vi "Vision Processing.vi"(4 "error in (no error)":errorcluster, 7 "Image Size":T3=enum."160x120") -> ()   [LabVIEW 2015]
doc: "This VI runs in parallel to other tasks. It gets images from the camera, processes them for color or shape and use that information to affect robot behavior."
uses:
  <vilib>/Rock Robotics/WPI/Camera/WPI_CameraImageSize.ctl
  <vilib>/Rock Robotics/WPI/Camera/WPI_CameraWhite Balance Values.ctl
  <vilib>/Rock Robotics/WPI/Camera/WPI_CameraExposure Values.ctl
  <vilib>/Rock Robotics/WPI/Camera/WPI_CameraFrameRate.ctl
  <vilib>/Rock Robotics/Network Tables/NT Read Number.vi
  Robot Global Data.vi
  <vilib>/vision/NI_Vision_Development_Module.lvlib
panel:
  in  "Blue or Luma or Val or Inten Range":cluster{"Lower value":i32, "Upper value":i32}={"Lower value"=0, "Upper value"=200}
  in  "Green or Sat Range":cluster{"Lower value":i32, "Upper value":i32}={"Lower value"=20, "Upper value"=230}
  in  "Red or Hue Range":cluster{"Lower value":i32, "Upper value":i32}={"Lower value"=150, "Upper value"=255}
  out "Image Dst Out 2":T1(plugin-control)
  in  "Operation":T2(ring)
  out "Particle Reports (Pixels)[0].Center of Mass":cluster{"X":dbl, "Y":dbl}={"X"=88.72549019607843, "Y"=42.09313725490196}
  out "Image Dst Out":T1(plugin-control)
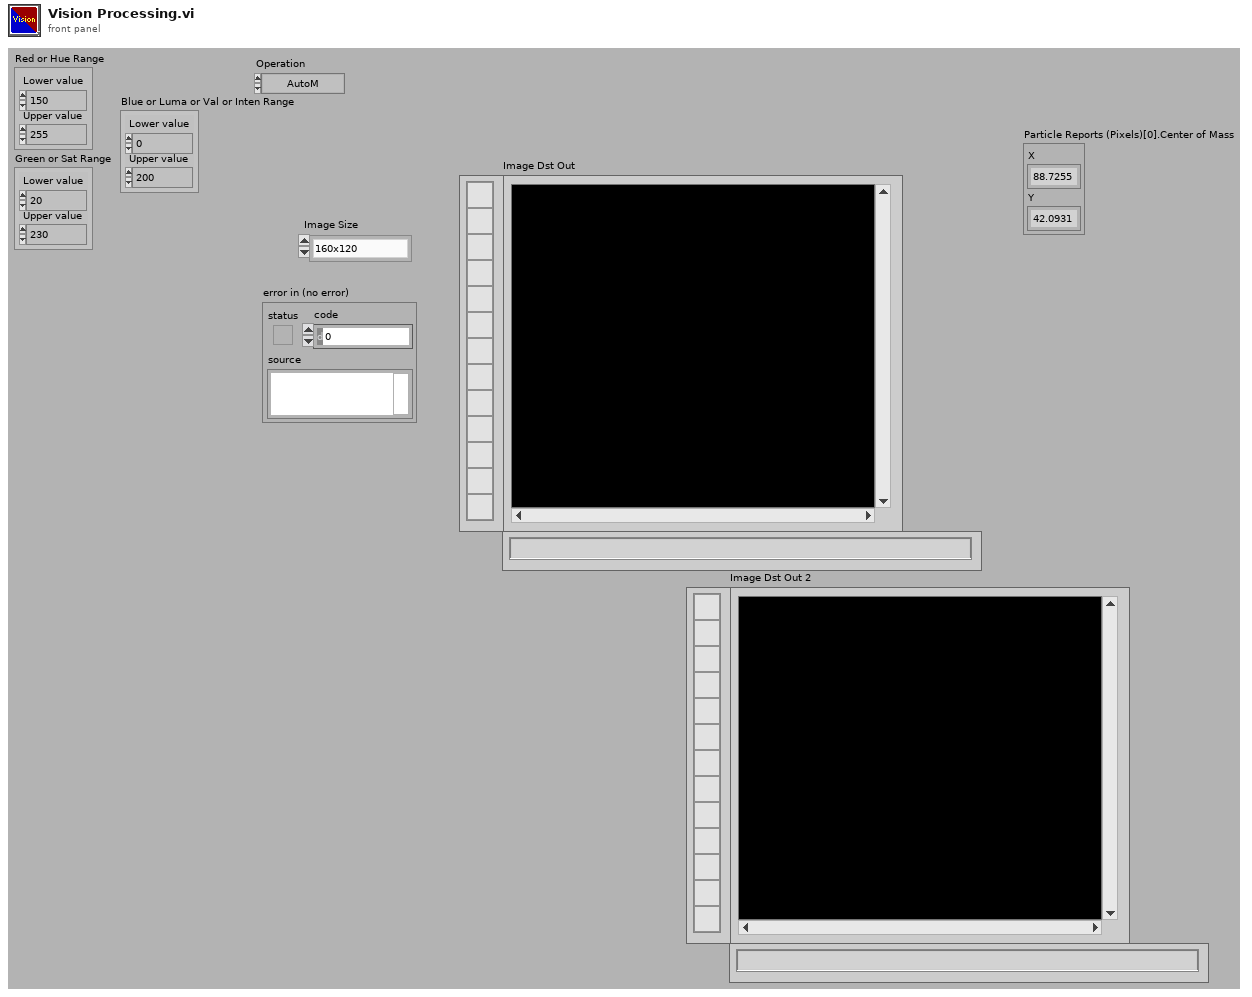
[diagram p1: front panel]
types:
  T1 = typedef "IMAQ Image.ctl" = refnum<image>
  T2 = enum32{"AutoM", "Close", "Dilate", "Erode", "Gradient", "Gradient out", "Gradient in", "Hit miss", "Open", "PClose", "POpen", "Thick", "Thin"}
  T3 = typedef "WPI_CameraImageSize.ctl" = enum16{"640x480", "320x240", "160x120", "Custom"}
  T4 = typedef "Image Type" = u32
  T5 = typedef "WPI_CameraFrameRate.ctl" = u32
  T6 = typedef "WPI_CameraExposure Values.ctl" = enum16{"Auto", "Flicker-free 50 Hz", "Flicker-free 60 Hz", "Hold current", "Custom"}
  T7 = typedef "WPI_CameraWhite Balance Values.ctl" = enum16{"Auto", "Fixed indoor", "Fixed outdoor 1", "Fixed outdoor 2", "Fixed fluorescent 1", "Fixed fluorescent 2", "Hold current", "Custom"}
  T8 = typedef "WPI_CameraDevRef.ctl" = cluster{"Camera Address":string, "CameraStatus":errorcluster}
  T9 = cluster{"Area":dbl, "Number of Holes":dbl, "Bounding Rect":cluster{"Left":dbl, "Top":dbl, "Right":dbl, "Bottom":dbl}, "Center of Mass":cluster{"X":dbl, "Y":dbl}, "Orientation":dbl, "Dimensions":cluster{"Width":dbl, "Height":dbl}}[]
  T10 = cluster{"Particle Reports (Pixels)[0]":cluster{"Area":dbl, "Number of Holes":dbl, "Bounding Rect":cluster{"Left":dbl, "Top":dbl, "Right":dbl, "Bottom":dbl}, "Center of Mass":cluster{"X":dbl, "Y":dbl}, "Orientation":dbl, "Dimensions":cluster{"Width":dbl, "Height":dbl}}, "Particle Reports (Pixels)[1]":cluster{"Area":dbl, "Number of Holes":dbl, "Bounding Rect":cluster{"Left":dbl, "Top":dbl, "Right":dbl, "Bottom":dbl}, "Center of Mass":cluster{"X":dbl, "Y":dbl}, "Orientation":dbl, "Dimensions":cluster{"Width":dbl, "Height":dbl}}, "Particle Reports (Pixels)[2]":cluster{"Area":dbl, "Number of Holes":dbl, "Bounding Rect":cluster{"Left":dbl, "Top":dbl, "Right":dbl, "Bottom":dbl}, "Center of Mass":cluster{"X":dbl, "Y":dbl}, "Orientation":dbl, "Dimensions":cluster{"Width":dbl, "Height":dbl}}, "Particle Reports (Pixels)[3]":cluster{"Area":dbl, "Number of Holes":dbl, "Bounding Rect":cluster{"Left":dbl, "Top":dbl, "Right":dbl, "Bottom":dbl}, "Center of Mass":cluster{"X":dbl, "Y":dbl}, "Orientation":dbl, "Dimensions":cluster{"Width":dbl, "Height":dbl}}, "Particle Reports (Pixels)[4]":cluster{"Area":dbl, "Number of Holes":dbl, "Bounding Rect":cluster{"Left":dbl, "Top":dbl, "Right":dbl, "Bottom":dbl}, "Center of Mass":cluster{"X":dbl, "Y":dbl}, "Orientation":dbl, "Dimensions":cluster{"Width":dbl, "Height":dbl}}, "Particle Reports (Pixels)[5]":cluster{"Area":dbl, "Number of Holes":dbl, "Bounding Rect":cluster{"Left":dbl, "Top":dbl, "Right":dbl, "Bottom":dbl}, "Center of Mass":cluster{"X":dbl, "Y":dbl}, "Orientation":dbl, "Dimensions":cluster{"Width":dbl, "Height":dbl}}, "Particle Reports (Pixels)[6]":cluster{"Area":dbl, "Number of Holes":dbl, "Bounding Rect":cluster{"Left":dbl, "Top":dbl, "Right":dbl, "Bottom":dbl}, "Center of Mass":cluster{"X":dbl, "Y":dbl}, "Orientation":dbl, "Dimensions":cluster{"Width":dbl, "Height":dbl}}, "Particle Reports (Pixels)[7]":cluster{"Area":dbl, "Number of Holes":dbl, "Bounding Rect":cluster{"Left":dbl, "Top":dbl, "Right":dbl, "Bottom":dbl}, "Center of Mass":cluster{"X":dbl, "Y":dbl}, "Orientation":dbl, "Dimensions":cluster{"Width":dbl, "Height":dbl}}, "Particle Reports (Pixels)[8]":cluster{"Area":dbl, "Number of Holes":dbl, "Bounding Rect":cluster{"Left":dbl, "Top":dbl, "Right":dbl, "Bottom":dbl}, "Center of Mass":cluster{"X":dbl, "Y":dbl}, "Orientation":dbl, "Dimensions":cluster{"Width":dbl, "Height":dbl}}}
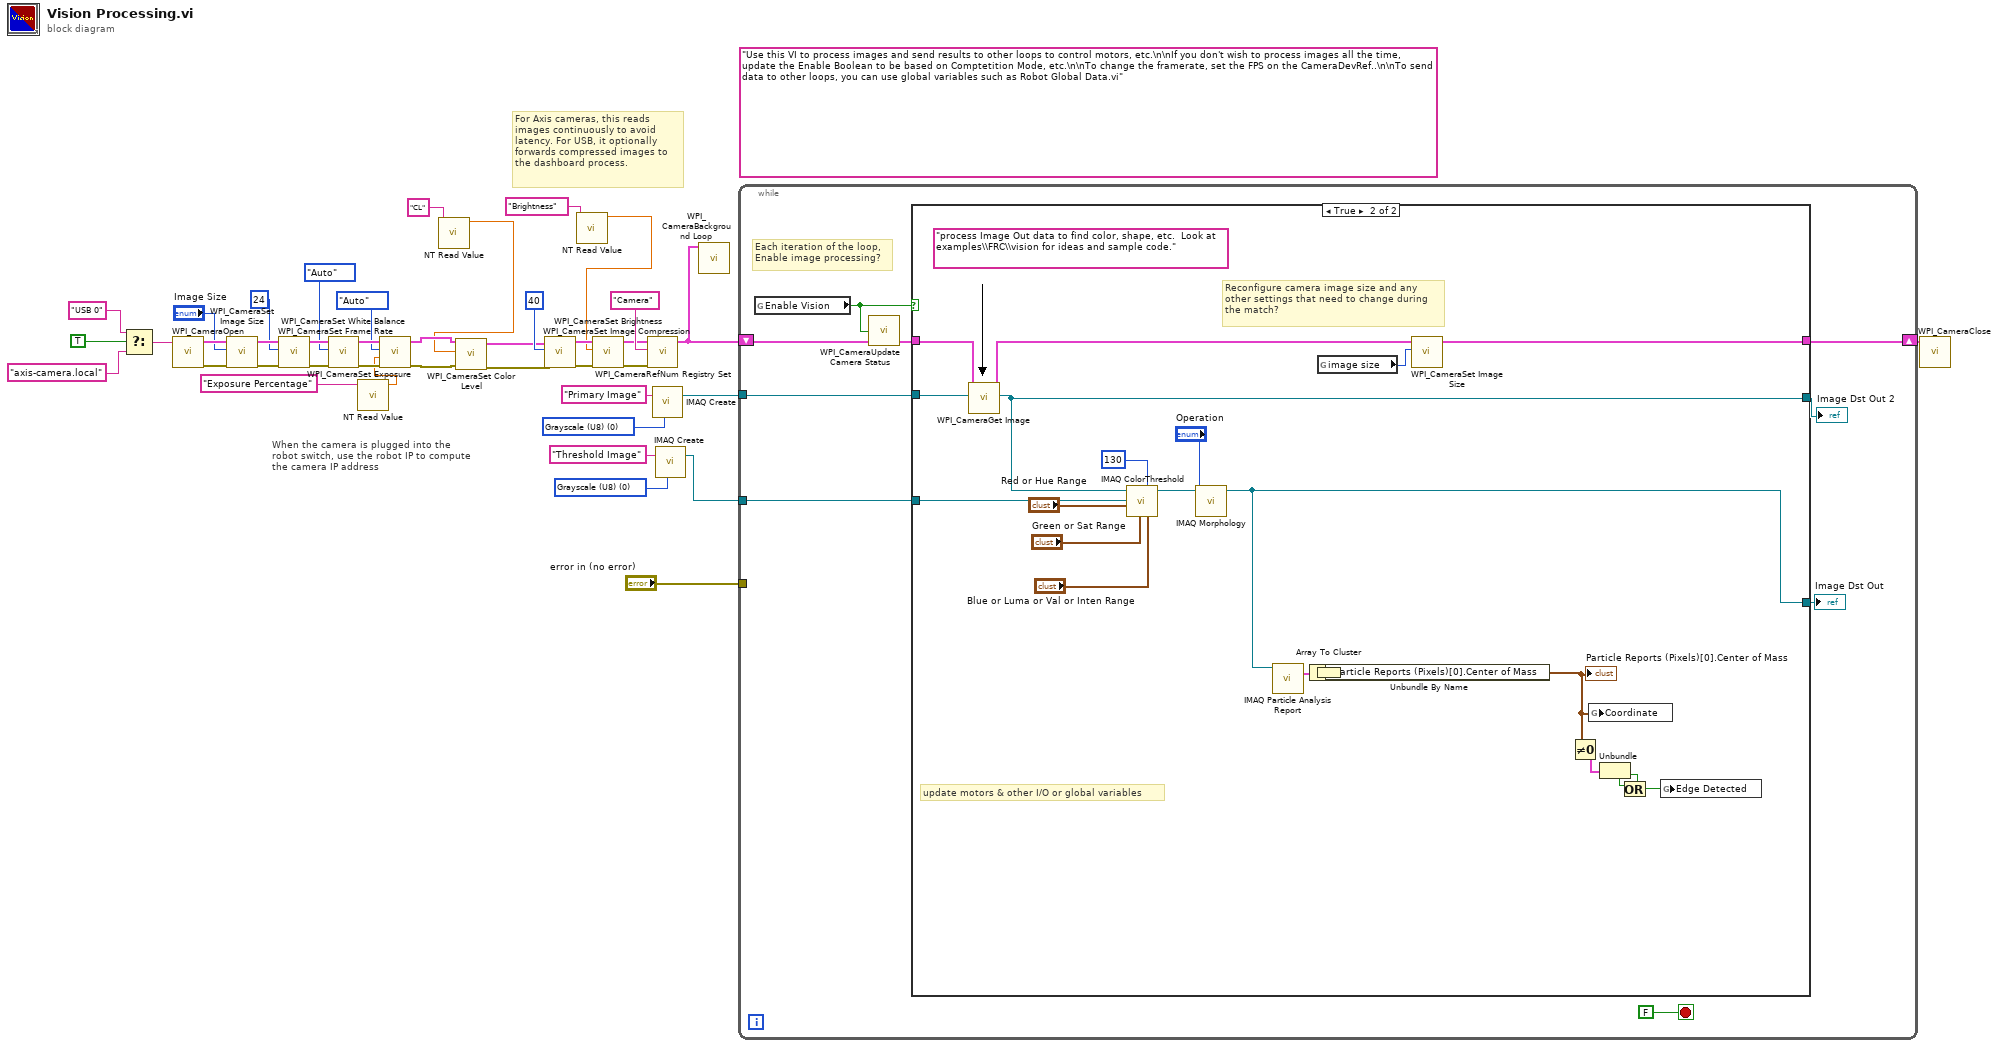
[diagram p0: block diagram]
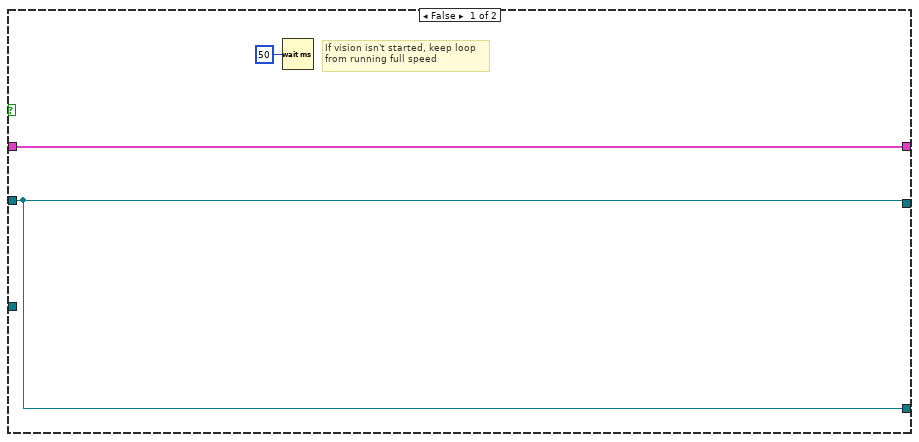
[diagram p2: hidden frame]
diagram:
  w13 = T4 0 items=["Grayscale (U8)", "Grayscale (I16)", "Grayscale (SGL)", "Complex (CSG)", "RGB (U32)", "HSL (U32)", "RGB (U64)", "Grayscale (U16)"] ("Image Type")
  (unwired) "Use this VI to process images and send results to other loops to control motors, etc.\n\nIf you don't wish to process images all the time, update the Enable Boolean to be based on Comptetition Mode, etc.\n\nTo change the framerate, set the FPS on the CameraDevRef..\n\nTo send data to other loops, you can use global variables such as Robot Global Data.vi"
  w41 = T4 0 items=["Grayscale (U8)", "Grayscale (I16)", "Grayscale (SGL)", "Complex (CSG)", "RGB (U32)", "HSL (U32)", "RGB (U64)"] ("Image Type")
  # "When the camera is plugged into the\nrobot switch, use the robot IP to compute\nthe camera IP address"
  # "For Axis cameras, this reads\nimages continuously to avoid\nlatency. For USB, it optionally\nforwards compressed images to\nthe dashboard process."
  n1 = Select(t="USB 0" ("format string"), s=TRUE ("dot notation? (F)"), f="axis-camera.local" ("format string")) -> (s? t:f=w15:string)
  n2 = call <vilib>:"WPI_CameraOpen.vi"("Camera Address"=w15) -> ("error out"=w31:errorcluster, "CameraDevRef"=w32:T8)  [unwired: 1 in, 8 out]
  n3 = call <vilib>:"WPI_CameraSet Image Size.vi"("error in (no error)"=w31, "Image Size"="Image Size", "CameraDevRef"=w32) -> ("error out"=w30:errorcluster, "CameraDevRef Out"=w33:T8)  [unwired: 1 in, 6 out]
  n4 = call <vilib>:"WPI_CameraSet Frame Rate.vi"("error in (no error)"=w30, "Frame Rate (fps)"=T5 24, "CameraDevRef"=w33) -> ("error out"=w29:errorcluster, "CameraDevRef Out"=w35:T8)  [unwired: 7 out]
  n5 = call <vilib>:"WPI_CameraSet White Balance.vi"("error in (no error)"=w29, "White Balance"=WPI_CameraWhite_Balance_Values."Auto", "CameraDevRef"=w35) -> ("error out"=w28:errorcluster, "CameraDevRef Out"=w34:T8)  [unwired: 1 in, 6 out]
  n6 = call-poly <vilib>:"NT Read Value.vi"("Name"="Exposure Percentage") -> ("Numeric"=w2:dbl)  [unwired: 9 in, 1 out]
  n7 = call <vilib>:"WPI_CameraSet Exposure.vi"("error in (no error)"=w28, "Exposure (%)"=w2, "Exposure"=WPI_CameraExposure_Values."Auto", "CameraDevRef"=w34) -> ("error out"=w9:errorcluster, "CameraDevRef Out"=w10:T8)  [unwired: 6 out]
  n8 = call-poly <vilib>:"NT Read Value.vi"("Name"="CL") -> ("Numeric"=w5:dbl)  [unwired: 9 in, 1 out]
  n9 = call <vilib>:"WPI_CameraSet Color Level.vi"("error in (no error)"=w9, "Color Level"=w5, "CameraDevRef"=w10) -> ("error out"=w7:errorcluster, "CameraDevRef Out"=w8:T8)  [unwired: 7 in]
  n10 = call <vilib>:"WPI_CameraSet Image Compression.vi"("error in (no error)"=w7, "Compression"=40, "CameraDevRef"=w8) -> ("error out"=w27:errorcluster, "CameraDevRef Out"=w36:T8)  [unwired: 7 out]
  n11 = call-poly <vilib>:"NT Read Value.vi"("Name"="Brightness") -> ("Numeric"=w4:dbl)  [unwired: 9 in, 1 out]
  n12 = call <vilib>:"WPI_CameraSet Brightness.vi"("error in (no error)"=w27, "Brightness"=w4, "CameraDevRef"=w36) -> ("error out"=w25:errorcluster, "CameraDevRef Out"=w26:T8)  [unwired: 7 out]
  n13 = call <vilib>:"WPI_CameraRefNum Registry Set.vi"("error in (no error)"=w25, "refnum name"="Camera", "CameraDevRef"=w26) -> ("CameraDevRef"=w21:T8)  [unwired: 1 in, 7 out]
  n14 = call "IMAQ Create"("Image Name"="Primary Image", "Image Type"=w41) -> ("New Image"=w39:T1)  [unwired: 2 in, 2 out]
  n15 = call "IMAQ Create"("Image Name"="Threshold Image", "Image Type"=w13) -> ("New Image"=w11:T1)  [unwired: 3 in, 1 out]
  n16 = call <vilib>:"WPI_CameraBackground Loop.vi"("CameraDevRef"=w21) -> ()  [unwired: 11 in]
  n17 = while {
    shift-right: [w49] -> w19
    shift-left: w21 -> [w47]
    tunnel: w39 -> [w48]
    tunnel: "error in (no error)" -> [_]
    tunnel: w11 -> [w44]
    stop <- FALSE stop-if-true
    # "Each iteration of the loop,\nEnable image processing?"
    n18 = global read "Robot Global Data.vi" "Enable Vision"() -> (w45:bool)
    n19 = call <vilib>:"WPI_CameraUpdate Camera Status.vi"("CameraDevRef In"=w47, "Enable Vision"=w45) -> ("CameraDevRef Out"=w46:T8)  [unwired: 3 in]
    n20 = case shown="True" w45 {
      tunnel: w48 -> [w51 w73]
      tunnel: [w53 w74] -> w49
      tunnel: w46 -> [w53 w71]
      tunnel: w44 -> [_ w69]
      tunnel: [w51 w59] -> w43
      tunnel: [w51 w57] -> w42
      frame False {
        # "If vision isn't started, keep loop\nfrom running full speed"
        n21 = Wait (ms)(milliseconds to wait=u32 50) -> ()  [unwired: 1 out]
      }
      frame True {
        (unwired) "process Image Out data to find color, shape, etc.  Look at examples\\FRC\\vision for ideas and sample code."
        # "update motors & other I/O or global variables"
        # "Reconfigure camera image size and any\nother settings that need to change during\nthe match?"
        n22 = call <vilib>:"WPI_CameraGet Image.vi"("Image"=w73, "CameraDevRef"=w71) -> ("Image Out"=w57:T1, "CameraDevRef Out"=w70:T8)  [unwired: 1 in, 7 out]
        n23 = call "IMAQ ColorThreshold"("Blue or Luma or Val or Inten Range"="Blue or Luma or Val or Inten Range", "Replace Value"=130, "Green or Sat Range"="Green or Sat Range", "Red or Hue Range"="Red or Hue Range", "Image Dst"=w69, "Image Src"=w57) -> ("Image Dst Out"=w60:T1)  [unwired: 4 in, 1 out]
        n24 = call "IMAQ Morphology"("Operation"="Operation", "Image Src"=w60) -> ("Image Dst Out"=w59:T1)  [unwired: 8 in, 1 out]
        n25 = call "IMAQ Particle Analysis Report"("Image"=w59) -> ("Particle Reports (Pixels)"=w67:T9)  [unwired: 5 in, 5 out]
        n26 = Array To Cluster(array=w67) -> (cluster=w66:T10)
        n27 = Unbundle By Name(w66) -> ("Particle Reports (Pixels)[0].Center of Mass"=w65:cluster{"X":dbl, "Y":dbl})
        "Particle Reports (Pixels)[0].Center of Mass" <- w65
        n28 = global read "Robot Global Data.vi" "image size"() -> (w72:T3)
        n29 = call <vilib>:"WPI_CameraSet Image Size.vi"("Image Size"=w72, "CameraDevRef"=w70) -> ("CameraDevRef Out"=w74:T8)  [unwired: 2 in, 7 out]
        n30 = Not Equal To 0?(x=w65) -> (x != 0?=w64:cluster{"X":bool, "Y":bool})
        n31 = global write "Robot Global Data.vi" "Coordinate"(w65) -> ()
        n32 = Unbundle(w64) -> ("X"=w63:bool, "Y"=w62:bool)
        n33 = Or(x=w63, y=w62) -> (x .or. y?=w61:bool)
        n34 = global write "Robot Global Data.vi" "Edge Detected"(w61) -> ()
      }
    }
    "Image Dst Out" <- w43
    "Image Dst Out 2" <- w42
  }
  n35 = call <vilib>:"WPI_CameraClose.vi"("CameraDevRef"=w19) -> ()  [unwired: 1 in, 10 out]
